vi "mqttBrokerRead.vi"(0 "mqtt in":refnum<class "mqtt.lvclass">, 11 "error in (no error)":errorcluster) -> (4 "mqtt out":refnum<class "mqtt.lvclass">, 6 "broker":T1, 15 "error out":errorcluster)   [LabVIEW 2017, in "mqtt.lvclass"]
uses:
  mqtt.lvclass
  mqttTypedef/mqttBroker.ctl
  mqtt.lvclass/mqtt.ctl
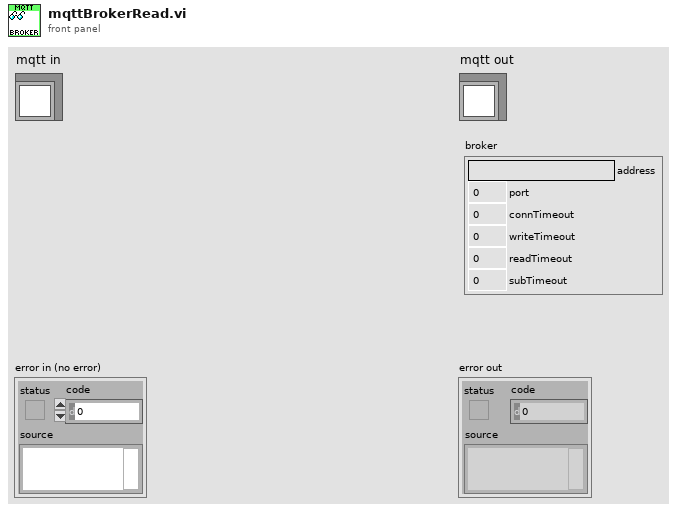
[diagram p1: front panel]
types:
  T1 = typedef "mqttBroker.ctl" = cluster{"address":string, "port":u16, "connTimeout":i32, "writeTimeout":i32, "readTimeout":i32, "subTimeout":i32}
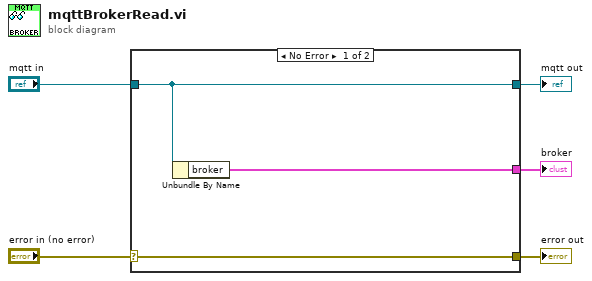
[diagram p0: block diagram]
diagram:
  n1 = case shown="No Error" "error in (no error)" {
    selector: "error in (no error)" -> [w8 w9]
    tunnel: [w8 w9] -> w4
    tunnel: [w7 w10] -> w2
    tunnel: "mqtt in" -> [w7 w10]
    tunnel: [w6 _] -> w1
    frame No Error {
      n2 = Unbundle By Name(w7) -> ("broker"=w6:T1)
    }
    frame Error {
    }
  }
  "error out" <- w4
  "mqtt out" <- w2
  "broker" <- w1
